vi "test_harness_fgm_partial_pipeline.vi"() -> ()   [LabVIEW 2017]
uses:
  quadProgControls/quadProgParams.ctl
  <vilib>/rvi/Emulation/niFpgaEmulationIsFPGAContextNoSignature.vi
  <vilib>/rvi/DataTransferAndStorage/Container/Common/niFpgaContainerGetUniqueNameForEmu.vi
  <vilib>/rvi/Memory/Memory_Emulation/niFpgaMemoryEmulationCacheClearOnFirstRun.vi
  <vilib>/rvi/Memory/Memory_Emulation/nirvimemoryEmulationManagerCache_MakeExclusive.vi
  <vilib>/rvi/Memory/Memory_Emulation/niFpgaMemoryEmulationValidateCache.vi
  <vilib>/rvi/Memory/Memory_Emulation/nirvimemoryEmulationManagerCache_InsertValue.vi
  <vilib>/Utility/error.llb/Clear Errors.vi
  <vilib>/rvi/Memory/Memory_Emulation/nirvimemoryEmulationManagerCache_ReleaseExclusive.vi
  <vilib>/rvi/Memory/Memory_Emulation/nirvimemoryEmulationManagerCache_GetValue.vi
  <vilib>/rvi/Memory/Memory_Emulation/nirvimemoryEmulationManagerCache_SetValue.vi
  <vilib>/rvi/Emulation/niFpgaProcessEmulError.vi
  <vilib>/rvi/Emulation/niFpgaSctlEmulationGetInTimedLoop.vi
  <vilib>/rvi/Memory/Memory_Emulation/nirvimemoryFastEmulation.vi
  <vilib>/rvi/Memory/Memory_Emulation/nirvimemoryEmulation.vi
  <vilib>/rvi/errors/nirviReportUnexpectedCaseInternalError (U32).vi
  <vilib>/rvi/DataTransferAndStorage/Container/XNode/niFpgaContainer.xnode
  <vilib>/rvi/DataTransferAndStorage/Register/Emulation/niFpgaRegisterEmulation.vi
panel:
  in  "idx2":i16=15
  in  "idx1":i16
  out "idx1":fxp<+/-,32,6>[](array[numeric])
  out "idx2":fxp<+/-,32,6>[](array[numeric])
  in  "z0":fxp<+/-,32,3>[](array[numeric])=[0.0, 0.0, 0.0, 0.0, 0.0, 0.0, 0.0, 0.0, 0.0, 0.0, 0.0, 0.0]
  in  "y0":fxp<+/-,32,3>[](array[numeric])=[0.0, 0.0, 0.0, 0.0, 0.0, 0.0, 0.0, 0.0, 0.0, 0.0, 0.0, 0.0]
  out "y":fxp<+/-,32,6>[](array[numeric])
  out "z":fxp<+/-,32,6>[](array[numeric])
  out "delta u(k)":fxp<+/-,32,3>
  in  "QP_params":T1={"maxIter"=0, "nuN"=24, "Ns_mpc"=0, "-beta"=-0.9987945556640625, "beta+1"=1.9987945556640625, "SLMAX"=0.039999961853027344}
  in  "big_mat_data":fxp<+/-,32,3>[](array[numeric])=[0.0, 0.0, 0.0, 0.0, 0.0, 0.0, 0.0, 0.0, 0.0, 0.0, 0.0, 0.0]
  in  "x":fxp<+/-,32,6>[](array[numeric])=[0.0, 0.0, 0.0, 0.0, 0.0, 0.0, 0.0, 0.0, 0.0, 0.0, 0.0, 0.0, 0.0, 0.0, 0.0, 0.0, 0.0, 0.0, 0.0, 0.0, 0.0, 0.0, 0.0, 0.0, 0.0]
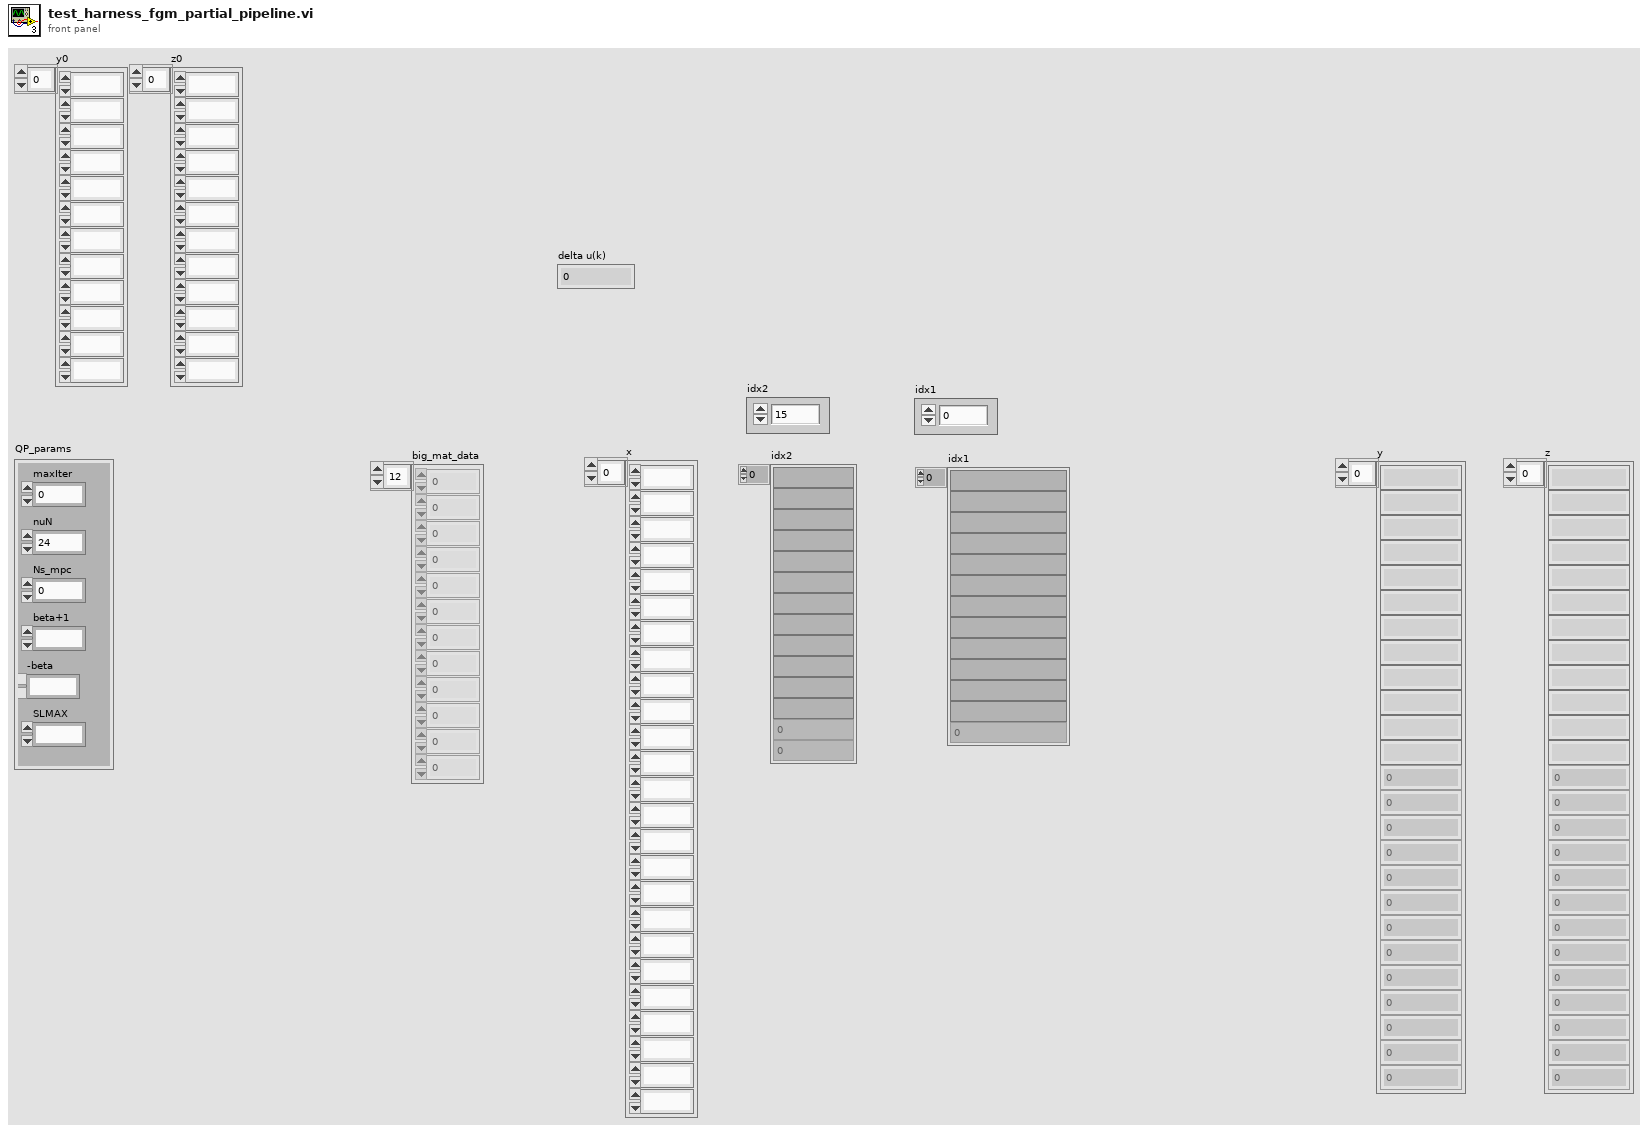
[diagram p1: front panel]
types:
  T1 = typedef "quadProgParams.ctl" = cluster{"maxIter":u16, "nuN":u16, "Ns_mpc":u16, "-beta":fxp<+/-,18,2>, "beta+1":fxp<+/-,18,2>, "SLMAX":fxp<+/-,18,-2>}
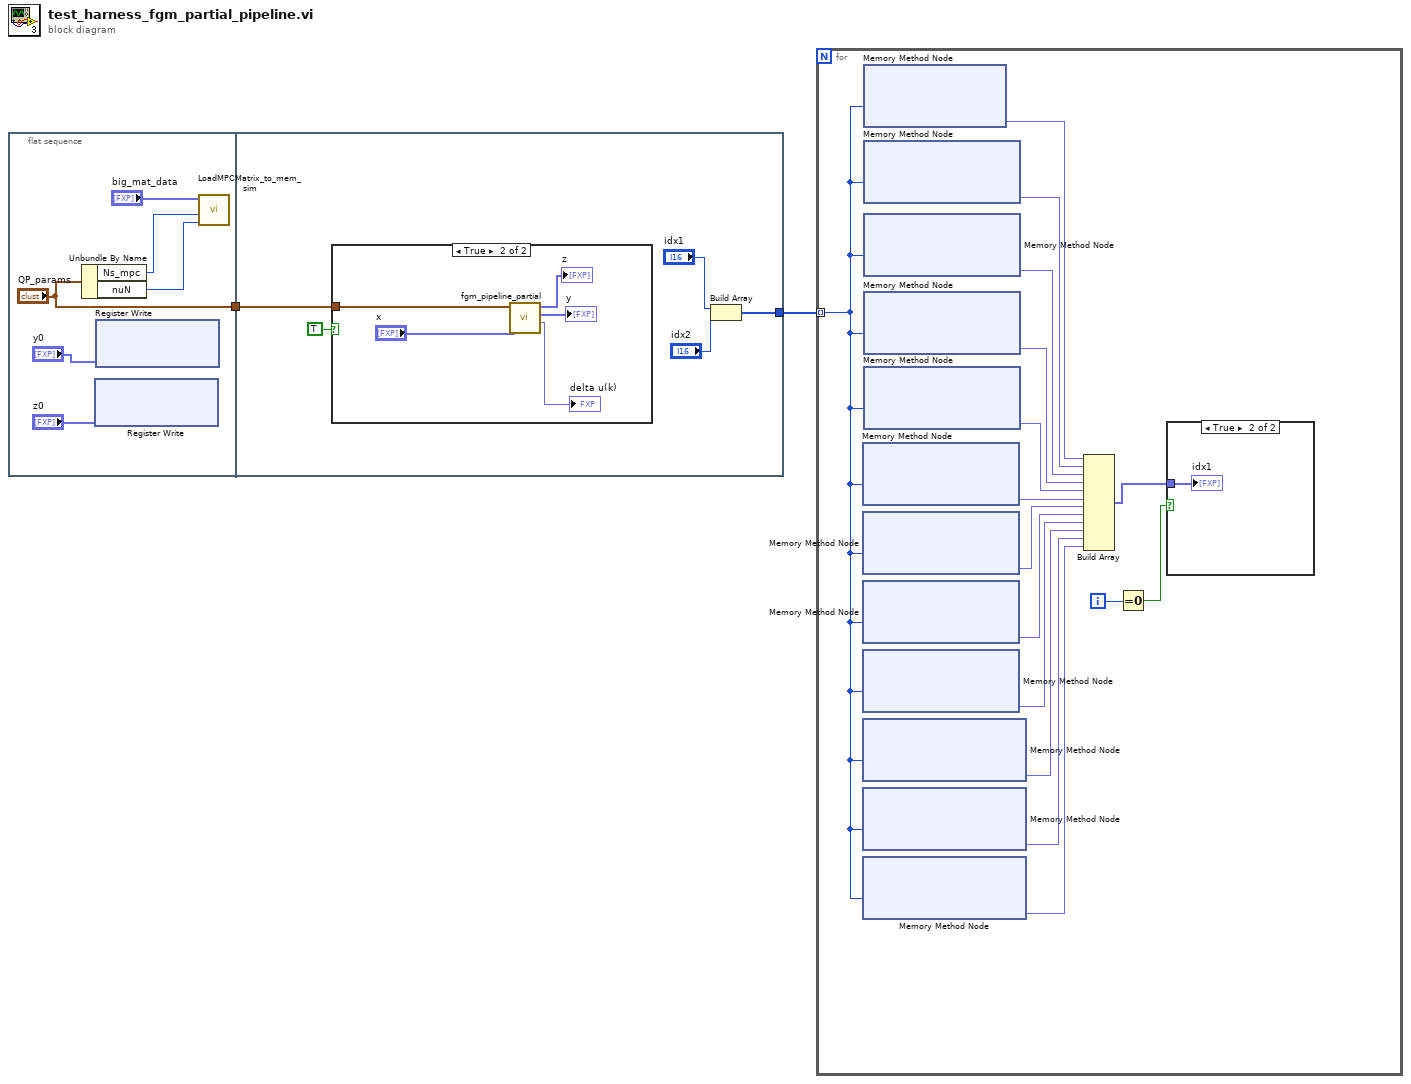
[diagram p0: block diagram]
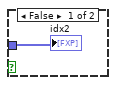
[diagram p3: hidden frame]
diagram:
  n1 = flat-sequence {
    tunnel: ["QP_params"] -> w1
    tunnel: [w13] -> w2
    tunnel: w1 -> [w12]
    frame #0 {
      n2 = Unbundle By Name("QP_params") -> ("Ns_mpc"=w3:u16, "nuN"=w6:u16)
      n3 = xnode ("Register Write")("Data"="z0") -> ()  [unwired: 1 in, 1 out]
      n4 = xnode ("Register Write")("Data"="y0") -> ()  [unwired: 1 in, 1 out]
      n5 = call "LoadMPCMatrix_to_mem_sim.vi"("nuN_mpc"=w6, "Ns"=w3, "big_mat_data"="big_mat_data") -> ()  [unwired: 9 in]
    }
    frame #1 {
      n6 = case shown="True" TRUE {
        tunnel: w12 -> [_ w14]
        frame False {
        }
        frame True {
          n7 = call "fgm_pipeline_partial.vi"("x_vec"="x", "QP_params"=w14) -> ("delta u(k)"=→"delta u(k)":fxp<+/-,32,3>, "y"=→"y":fxp<+/-,32,6>[], "z"=→"z":fxp<+/-,32,6>[])  [unwired: 7 in]
        }
      }
      n8 = Build Array("idx1", "idx2") -> (w13:i16[])
    }
  }
  n9 = for {
    tunnel: w2 -> [w34] mode=indexing
    i -> [w19]
    n10 = xnode ("Memory Method Node")("Address"=w34) -> ("Data"=w28:fxp<+/-,32,2>)  [unwired: 1 in, 1 out]
    n11 = xnode ("Memory Method Node")("Address"=w34) -> ("Data"=w27:fxp<+/-,32,2>)  [unwired: 1 in, 1 out]
    n12 = xnode ("Memory Method Node")("Address"=w34) -> ("Data"=w26:fxp<+/-,32,2>)  [unwired: 1 in, 1 out]
    n13 = xnode ("Memory Method Node")("Address"=w34) -> ("Data"=w25:fxp<+/-,32,2>)  [unwired: 1 in, 1 out]
    n14 = xnode ("Memory Method Node")("Address"=w34) -> ("Data"=w24:fxp<+/-,32,2>)  [unwired: 1 in, 1 out]
    n15 = xnode ("Memory Method Node")("Address"=w34) -> ("Data"=w23:fxp<+/-,32,2>)  [unwired: 1 in, 1 out]
    n16 = xnode ("Memory Method Node")("Address"=w34) -> ("Data"=w22:fxp<+/-,32,2>)  [unwired: 1 in, 1 out]
    n17 = xnode ("Memory Method Node")("Address"=w34) -> ("Data"=w33:fxp<+/-,32,2>)  [unwired: 1 in, 1 out]
    n18 = xnode ("Memory Method Node")("Address"=w34) -> ("Data"=w32:fxp<+/-,32,2>)  [unwired: 1 in, 1 out]
    n19 = xnode ("Memory Method Node")("Address"=w34) -> ("Data"=w31:fxp<+/-,32,2>)  [unwired: 1 in, 1 out]
    n20 = xnode ("Memory Method Node")("Address"=w34) -> ("Data"=w30:fxp<+/-,32,2>)  [unwired: 1 in, 1 out]
    n21 = xnode ("Memory Method Node")("Address"=w34) -> ("Data"=w29:fxp<+/-,32,2>)  [unwired: 1 in, 1 out]
    n22 = Build Array(w33, w32, w31, w30, w29, w28, w27, w26, w25, w24, w23, w22) -> (w20:fxp<+/-,32,2>[])
    n23 = Equal To 0?(x=w19) -> (x = 0?=w21:bool)
    n24 = case shown="True" w21 {
      tunnel: w20 -> [w35 w36]
      frame False {
        "idx2" <- w35
      }
      frame True {
        "idx1" <- w36
      }
    }
  }
